vi "Set Live Current.vi"(8 "error in":errorcluster, 10 "I":sgl, 11 "TEC 1090 in":refnum<class "Meerstetter TEC.lvclass">) -> (0 "error out":errorcluster, 3 "TEC 1090 out":refnum<class "Meerstetter TEC.lvclass">)   [LabVIEW 2014, in "Meerstetter Lib.lvlib" / "Meerstetter TEC.lvclass"]
uses:
  Meerstetter TEC.lvclass
  reusable/Session APIs/Serial/Serial Session.lvclass
  Meerstetter TEC.lvclass/Meerstetter TEC.ctl
  Configurable Device/Configurable Device.lvclass/Configurable Device.ctl
  Accessors/Read SerialSession.vi
  Configurable Device/Read Log Session.vi
  Configurable Device/Read ID.vi
  reusable/Session APIs/Serial/Public/Asynchronous Write.vi
  reusable/Session APIs/Serial/Public/Asynchronous Read.vi
  <userlib>/_Session Fwk/Session - Root.lvclass
  reusable/Session APIs/Session Log/System Log.lvclass
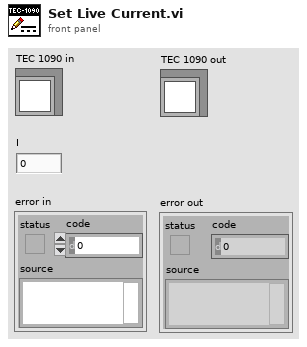
[diagram p1: front panel]
types:
  T1 = typedef "Session - Root.lvclass/Session Handle.ctl" = refnum<data-value>
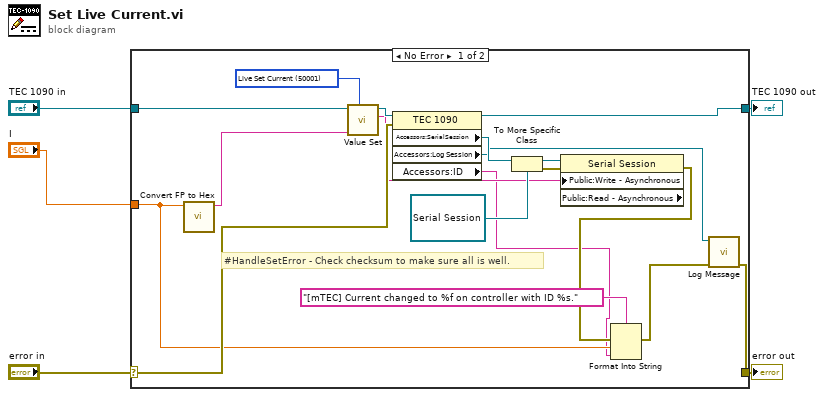
[diagram p0: block diagram]
diagram:
  n1 = case shown="No Error" "error in" {
    selector: "error in" -> [w19 w25]
    tunnel: [w6 w25] -> w4
    tunnel: [w14 w24] -> w2
    tunnel: "TEC 1090 in" -> [w23 w24]
    tunnel: "I" -> [w12 _]
    frame No Error {
      w21 = u16 50001 items=["Input Selection"=2000, "Status"=2010, "Set Current"=2020, "Set Voltage"=2021, "Current Limitation"=2030, "Voltage Limitation"=2031, "Current Error Threshold"=2032, "Voltage Error Threshold"=2033, "Channel Baud Rate"=2050, "Response Delay"=2052, "Timeout"=2060, "Target Object Temperature"=3000, "Coarse Temp Ramp"=3003, "Proximity Width"=3002, "Kp"=3010, "Ti"=3011, "Td"=3012, "D Part Damping D1"=3013, "Live Enable"=50000, "Live Set Current"=50001, "Live Set Voltage"=50002, "Object Target Temperature"=50012, "Save Data to Flash"=108] ("Value Set")
      # "#HandleSetError - Check checksum to make sure all is well."
      n2 = call "Convert FP to Hex.vi"("Number"=w12) -> ("hex integer string"=w22:string)  [unwired: 10 in]
      n3 = call "Value Set.vi"("Value Set"=w21, "Value"=w22, "TEC 1090"=w23) -> ("hex integer string"=w13:string, "TEC 1091"=w20:refnum<class "Meerstetter TEC.lvclass">)  [unwired: 7 in]
      n4 = property class="TEC 1090"(reference=w20, error in=w19) -> (reference out=w14:refnum<class "Meerstetter TEC.lvclass">, "Accessors:SerialSession"=w18:T1, "Accessors:Log Session"=w8:T1, "Accessors:ID"=w7:string)  [unwired: 1 out]
      n5 = To More Specific Class(target class=refnum<data-value> refnum, reference=w18) -> (specific class reference=w16:refnum<data-value>, error out=w15:errorcluster)  [unwired: 1 in]
      n6 = property class="Serial Session" props=["Public:Write - Asynchronous", "Public:Read - Asynchronous"](reference=w16, error in=w15, "Public:Write - Asynchronous"=w13) -> (error out=w10:errorcluster)  [unwired: 2 out]
      n7 = Format Into String(format string="[mTEC] Current changed to %f on controller with ID %s.", error in=w10, w12, w7) -> (error out=w11:errorcluster)  [unwired: 1 in, 1 out]
      n8 = call "Log Message.vi"("error in"=w11, "session in"=w8) -> ("error out"=w6:errorcluster)  [unwired: 8 in, 1 out]
    }
    frame Error {
    }
  }
  "error out" <- w4
  "TEC 1090 out" <- w2
